vi "相机2图像处理.vi"(6 "生产统计3":T3, 10 "自动":bool, 11 "Img(in)":T2) -> (0 "生产统计3out":T3, 2 "3结果":bool=TRUE, 3 "Img(out)":T2(plugin-control))   [LabVIEW 2014]
uses:
  Controls/MsgAction.ctl
  Global.vi
  <vilib>/vision/Image Controls.llb/IMAQ Image.ctl
  Controls/ProductNum.ctl
panel:
  out "添加的数组":i32[](array[numeric])
  in  "显示坐标":cluster{dbl, "Numeric":dbl}[](array[cluster])=[{300.0, "Numeric"=200.0}, {300.0, "Numeric"=400.0}, {300.0, "Numeric"=600.0}, {300.0, "Numeric"=800.0}, {300.0, "Numeric"=1000.0}, {300.0, "Numeric"=1200.0}, {300.0, "Numeric"=1400.0}]
  out "存档数据":T1
  in  "Img Path 2":path=path "D:/雷迪埃存图/Cam3Img/2018-0930/Cam3Img2018-0930-174133.jpg"
  in  "error in":errorcluster
  # "%"
  # "%"
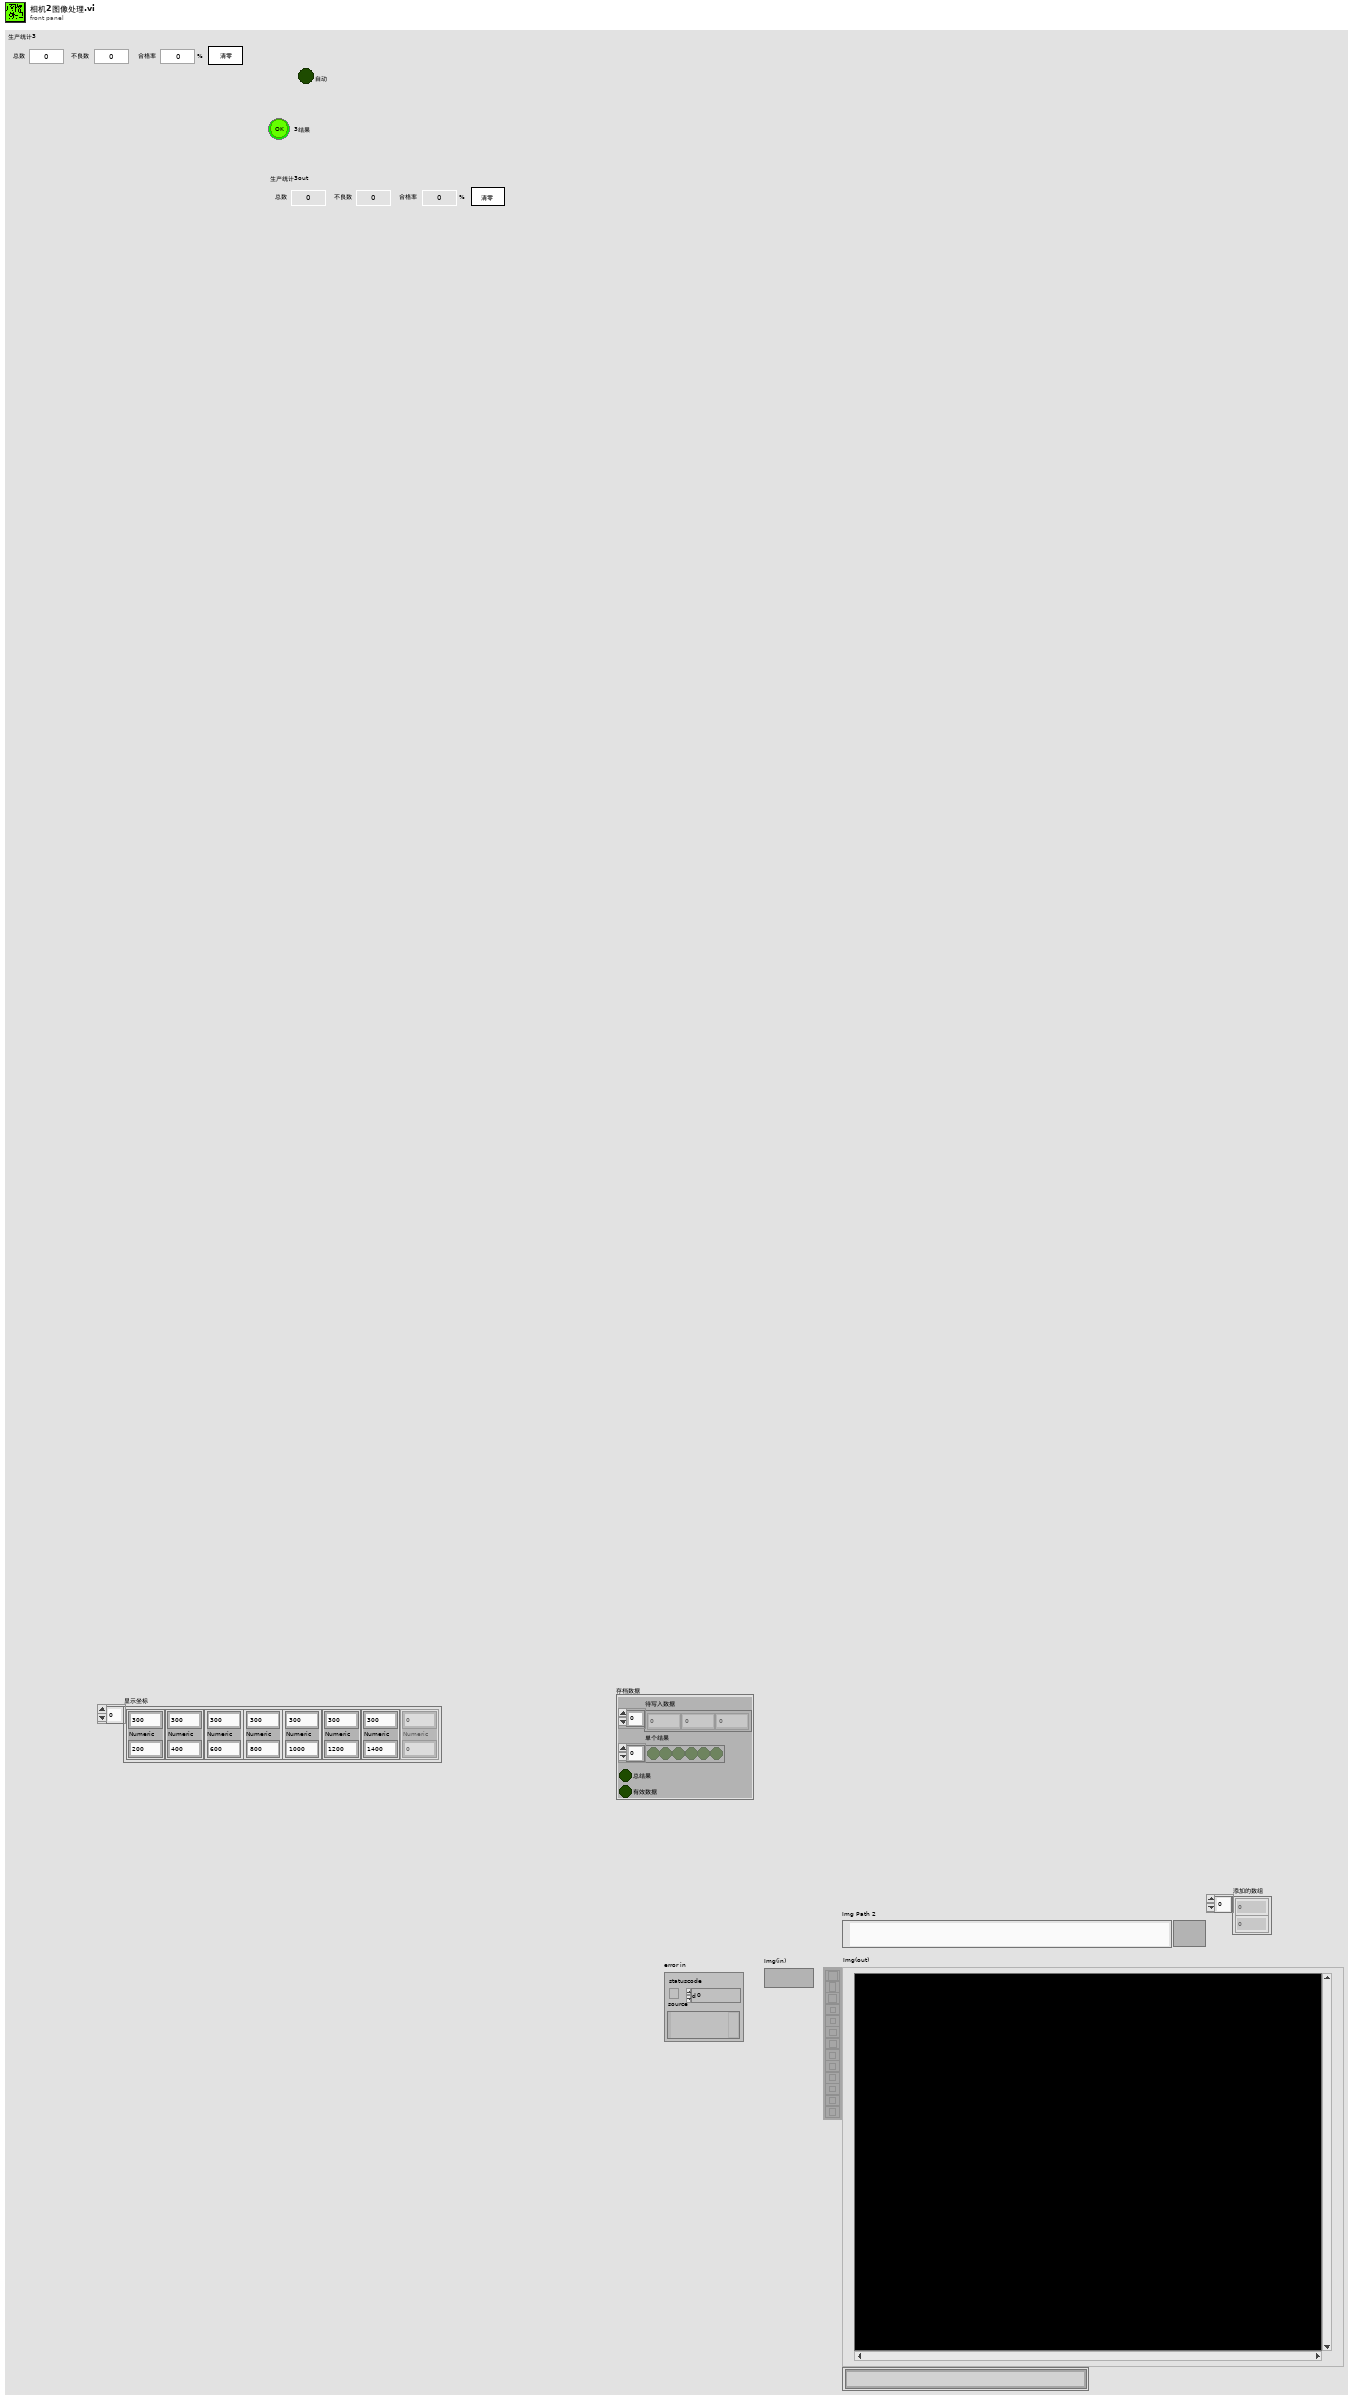
[diagram p1: front panel]
types:
  T1 = typedef "控件-存档数据和结果.ctl" = cluster{"待写入数据":dbl[], "单个结果":bool[], "总结果":bool, "有效数据":bool}
  T2 = typedef "IMAQ Image.ctl" = refnum<image>
  T3 = typedef "ProductNum.ctl" = cluster{"总数":u64, "不良数":u64, "合格率":dbl, "清零":bool}
  T4 = typedef "升立德IOAction.ctl" = enum16{"IO卡初始化", "读信号(16bit)", "写信号(16bit)", "写拍照Mark1完成信号OFF", "写拍照Mark1完成信号ON", "写拍照Mark2完成信号OFF", "写拍照Mark2完成信号ON", "写拍照PCB孔结果", "GetInfo", "清除目标"}
  T5 = typedef "MsgAction.ctl" = enum16{"初始化", "添加消息", "区分结果添加消息", "清空消息", "获取消息"}
  T6 = cluster{"Center (Pixels)":cluster{"X":sgl, "Y":sgl}, "Radius (Pixels)":dbl, "Center (Real-World)":cluster{"X":sgl, "Y":sgl}, "Radius (Real-World)":dbl, "Roundness (Real-World)":dbl, "Average Strength":dbl, "Average SNR (dB)":dbl}
  T7 = cluster{"Minimal Value":sgl, "Maximal Value":sgl, "Mean Value":sgl, "Standard  Variation":sgl, "Area (pixels)":i32}
  T8 = typedef "ModeEditeControl.ctl" = cluster{"AllModelFold":path, "AllModelNamePath":path, "所有零件型号":string[], "当前零件型号":string, "所有建立零件信息":string[][], "当前零件序号":i32, "当前产品信息":T9}
  T9 = typedef "ModelInfo.ctl" = cluster{"产品型号":string, "二维码拍照":u32, "Mark点拍照":u32}
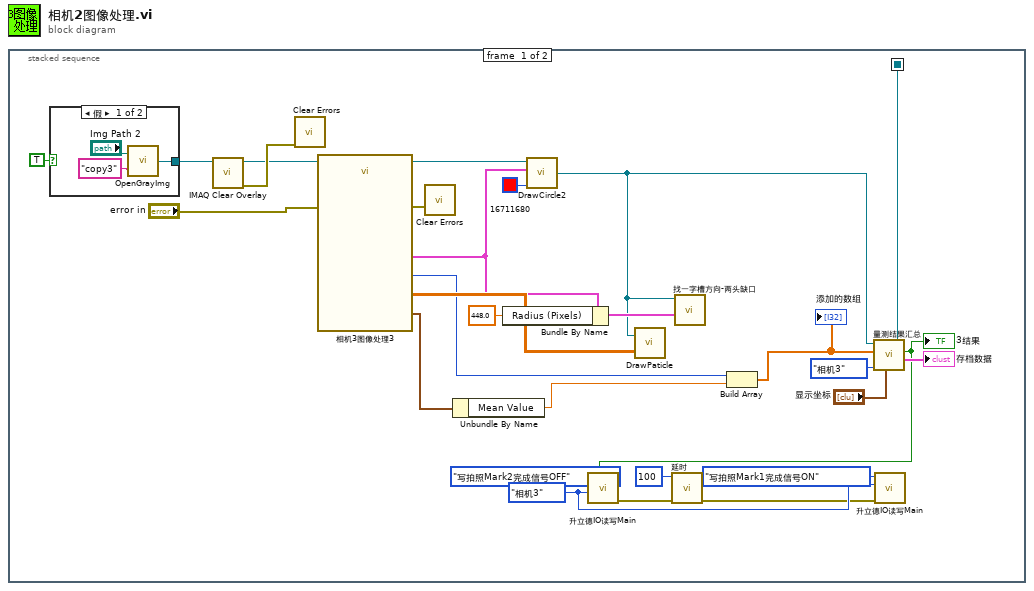
[diagram p0: block diagram]
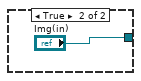
[diagram p2: hidden frame]
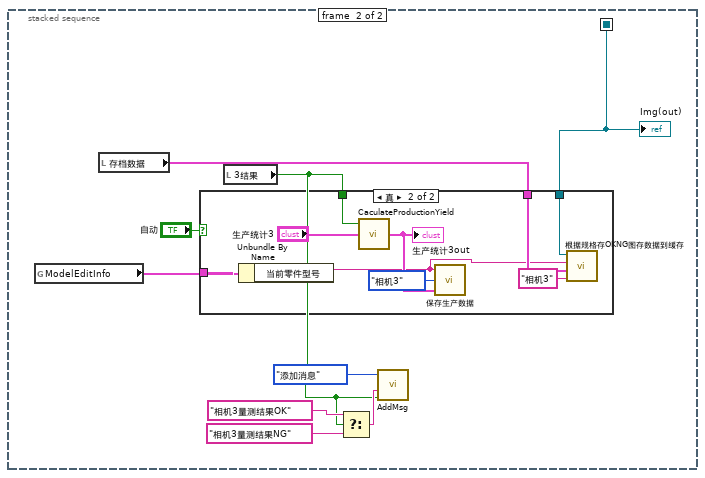
[diagram p3: hidden frame]
diagram:
  n1 = stacked-sequence {
    seq-local: [w8 _] -> [_ w35]
    frame #0 {
      w17 = enum16{"相机1", "相机2", "相机3", "相机4"}."相机3" ("选择相机")
      n2 = case shown="假" TRUE {
        tunnel: [w30 "Img(in)"] -> w27
        frame False {
          n3 = call "OpenGrayImg.vi"("Image Name"="copy3", "Img Path"="Img Path 2") -> ("Image Out"=w30:T2)
        }
        frame True {
        }
      }
      n4 = call "IMAQ Clear Overlay"("Image"=w27) -> ("error out"=w26:errorcluster, "Image Out"=w7:T2)  [unwired: 9 in]
      n5 = call <vilib>:"Clear Errors.vi"("error in (no error)"=w26) -> ()  [unwired: 5 in, 2 out]
      n6 = call "相机3图像处理3"("Image In"=w7, "error in"="error in") -> ("Image Out"=w22:T2, "Number of Particles (Particle Analysis 1)"=w3:i32, "Fitted Circle (Find Circular Edge 1)"=w5:T6, "Particle Measurements (Pixels) (Particle Analysis 1)"=w23:dbl[][], "Statistics (内导体有无安装)"=w2:T7, "error out"=w24:errorcluster)  [unwired: 20 in]
      n7 = call <vilib>:"Clear Errors.vi"("error in (no error)"=w24) -> ()  [unwired: 5 in, 2 out]
      n8 = Unbundle By Name(w2) -> ("Mean Value"=w1:sgl)
      n9 = Bundle By Name(cluster=w5, "Radius (Pixels)"=448.0) -> (w21:T6)
      n10 = call "DrawCircle2.vi"("Color"=u32 16711680, "Fitted Circle (左圆)"=w5, "Img in"=w22) -> ("Img out"=w11:T2)  [unwired: 1 in]
      n11 = call "DrawPaticle.vi"("Particle Measurements (Pixels) (左引脚)"=w23, "引用句柄输入"=w11) -> ()  [unwired: 1 out]
      n12 = call "找一字槽方向-两头缺口.vi"("Fitted Circle"=w21, "Img in"=w11) -> ()  [unwired: 7 in, 3 out]
      n13 = Build Array(w3, w1) -> (w13:sgl[])
      "添加的数组" <- w13
      n14 = call "量测结果汇总.vi"("显示坐标"="显示坐标", "选项"=enum16{"相机1", "相机2", "相机3", "相机4"}."相机3", "量测数据1维"=w13, "Img in"=w11) -> ("存档数据"=→"存档数据":T1, "结果"=w4:bool, "ImgOut"=w8:T2)  [unwired: 3 in]
      "3结果" <- w4
      n15 = call "升立德IO读写Main.vi"(7:w4, "选择相机"=w17, "选项"=升立德IOAction."写拍照Mark2完成信号OFF") -> ("error out"=w16:errorcluster)  [unwired: 4 in, 4 out]
      n16 = call "延时.vi"("错误in"=w16, "等待时间（毫秒）"=u32 100) -> ("错误in"=w15:errorcluster)  [unwired: 9 in]
      n17 = call "升立德IO读写Main.vi"("error in"=w15, "选择相机"=w17, "选项"=升立德IOAction."写拍照Mark1完成信号ON") -> ()  [unwired: 4 in, 5 out]
    }
    frame #1 {
      n18 = global read "Global.vi" "ModelEditInfo"() -> (w34:T8)
      n19 = local read "存档数据"() -> (w40:T1)
      n20 = local read "3结果"() -> (w33:bool)
      n21 = case shown="真" "自动" {
        tunnel: w33 -> [_ w49]
        tunnel: w40 -> [_ w45]
        tunnel: w35 -> [_ w44]
        tunnel: w34 -> [_ w43]
        frame False {
        }
        frame True {
          n22 = Unbundle By Name(w43) -> ("当前零件型号"=w42:string)
          n23 = call "CaculateProductionYield.vi"("生产统计"="生产统计3", "Result(in)"=w49) -> ("良率统计out"=w48:T3)  [unwired: 1 in]
          "生产统计3out" <- w48
          n24 = call "保存生产数据.vi"("良率统计"=w48, "选择拍照内容"=enum16{"相机1", "相机2", "相机3", "相机4"}."相机3" ("选择相机"), "产品型号"=w42) -> ()
          n25 = call "根据规格存OKNG图存数据到缓存.vi"("选择相机字符串"="相机3", "存档数据和结果"=w45, "当前零件型号"=w42, "Img输入"=w44) -> ()  [unwired: 8 in]
        }
      }
      n26 = Select(t="相机3量测结果OK" ("消息显示"), s=w33, f="相机3量测结果NG" ("消息显示")) -> (s? t:f=w38:string)
      n27 = call "AddMsg.vi"("Result"=w33, "添加消息"=w38, "消息Action"=MsgAction."添加消息") -> ()  [unwired: 1 in, 1 out]
      "Img(out)" <- w35
    }
  }
